vi "EnvFloMet.vi"() -> ()   [LabVIEW 2016]
uses:
  <vilib>/addons/database/NI_Database_API.lvlib
panel:
  in  "stop":bool
  out "error out":errorcluster
  in  "error in (no error)":errorcluster
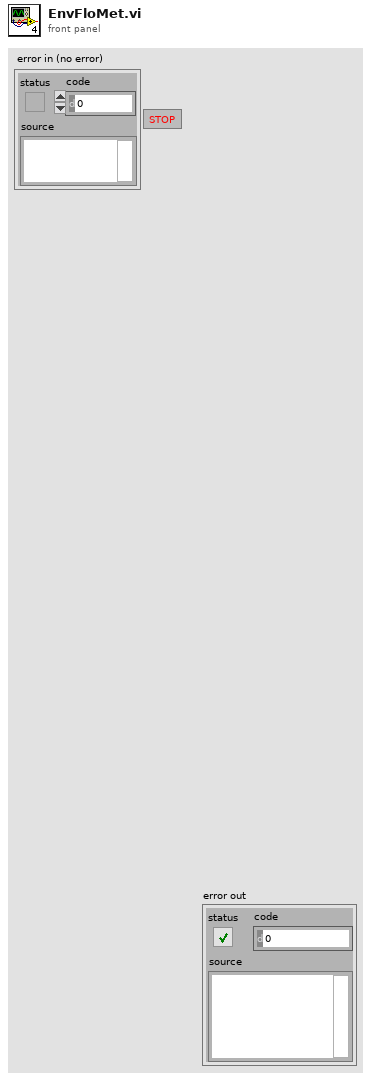
[diagram p1: front panel]
types:
  T1 = typedef "NI_Database_API.lvlib/Conn ObjectReference.ctl" = refnum<k1>
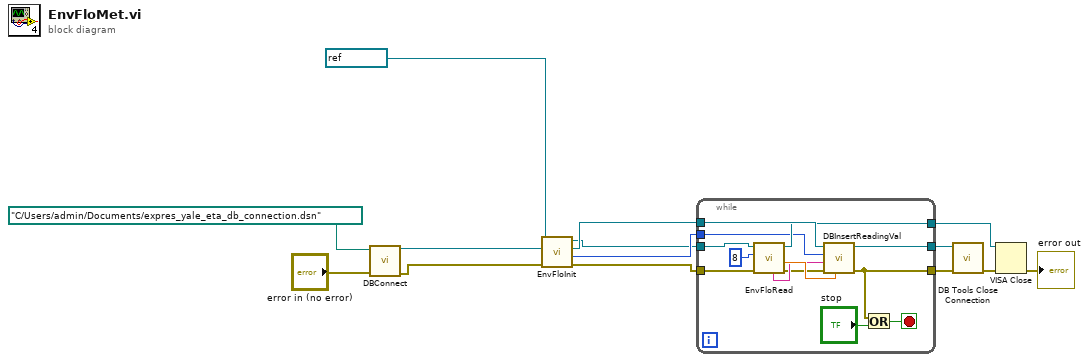
[diagram p0: block diagram]
diagram:
  n1 = call "DBConnect.vi"("error in (no error)"="error in (no error)", "connection path"=path "C:/Users/admin/Documents/expres_yale_eta_db_connection.dsn" ("connection information")) -> ("error out"=w12:errorcluster, "db connection out"=w1:T1)  [unwired: 8 in]
  n2 = call "EnvFloInit.vi"("error in (no error)"=w12, "db connection in"=w1, "VISA Refnum in"=refnum<visa-resource-name> "COM4") -> ("error out"=w5:errorcluster, "sensor id"=w8:i32, "db connection out"=w11:T1, "VISA Refnum out"=w4:refnum<visa-resource-name>)  [unwired: 5 in]
  n3 = while {
    tunnel: w8 -> [w15]
    tunnel: w5 -> [w25]
    tunnel: [w16] -> w9
    tunnel: w11 -> [w27]
    tunnel: [w26] -> w10
    tunnel: w4 -> [w24]
    tunnel: [w22] -> w3
    stop <- w17 stop-if-true
    n4 = call "EnvFloRead.vi"("error in (no error)"=w25, "read byte count"=u32 8, "VISA Refnum in"=w24) -> ("error out"=w19:errorcluster, "value"=w21:dbl, "VISA Refnum out"=w22:refnum<visa-resource-name>, "timestamp"=w20:string)  [unwired: 3 in, 2 out]
    n5 = call "DBInsertReadingVal.vi"("db connection in"=w27, "sensor id"=w15, "timestamp"=w20, "error in (no error)"=w19, "reading value"=w21) -> ("db connection out"=w26:T1, "error out"=w16:errorcluster)  [unwired: 4 in]
    n6 = Or(x=w16, y="stop") -> (x .or. y?=w17:bool)
  }
  n7 = call <vilib>:"DB Tools Close Connection.vi"("error in (no error)"=w9, "connection reference"=w10) -> ("error out"=w2:errorcluster)  [unwired: 5 in]
  n8 = VISA Close(VISA resource name=w3, error in (no error)=w2) -> (error out=→"error out":errorcluster)
